vi "Init BLRL Source.vi"(8 "error in (no error)":errorcluster, 10 "Config JSON":string, 11 "User BluelinesRedlines in":refnum<class "User BluelinesRedlines.lvclass">) -> (0 "error out":errorcluster, 3 "User BluelinesRedlines out":refnum<class "User BluelinesRedlines.lvclass">)   [LabVIEW 2020, in "VolatusGUIElements.lvlib" / "User BluelinesRedlines.lvclass"]
uses:
  User BluelinesRedlines.lvclass
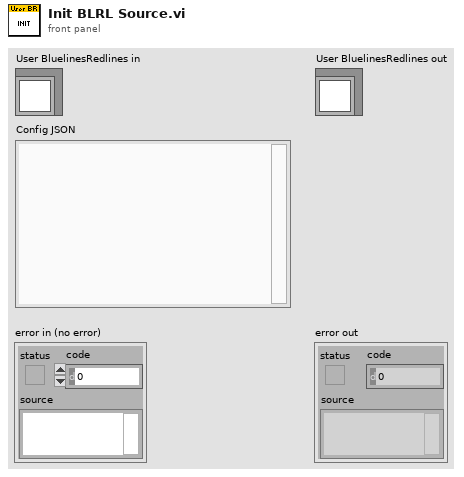
[diagram p1: front panel]
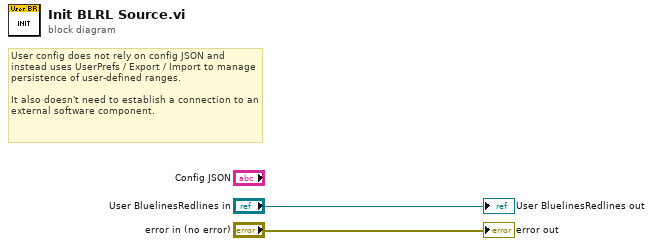
[diagram p0: block diagram]
diagram:
  # "User config does not rely on config JSON and instead uses UserPrefs / Export / Import to manage persistence of user-defined ranges.\n\nIt also doesn't need to establish a connection to an external software component."
  "error out" <- "error in (no error)"
  "User BluelinesRedlines out" <- "User BluelinesRedlines in"
